vi "Run Test.vi"(8 "error in (no error)":errorcluster, 11 "Example Test In":refnum<class "Program RF.lvclass">) -> (0 "error out":errorcluster, 1 "Fail Codes":string[](array[string]), 2 "Tests Passed":bool[](array[boolean]), 3 "Example Test Out":refnum<class "Program RF.lvclass">)   [LabVIEW 2015, in "Program RF.lvclass"]
uses:
  Program RF.lvclass
  Test Class/Test Class.lvclass/Test Class.ctl
  <userlib>/_OpenG.lib/array/array.llb/Filter 1D Array with Scalar (Boolean)__ogtk.vi
  Classes/Application/Class/Application.lvclass
  Test Class/Test Class.lvclass
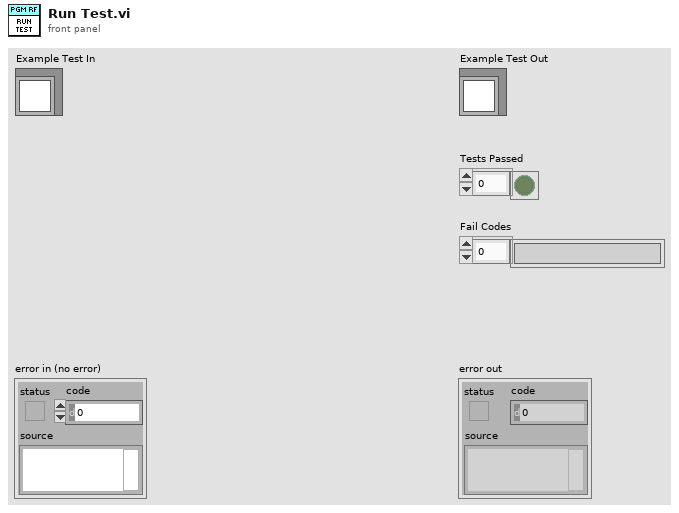
[diagram p1: front panel]
types:
  T1 = cluster{"status":bool, "code":i32, "source":string, "Position":u32}
  T2 = cluster{"Serial Number Reference":refnum<vi>, "Status Message Reference":refnum<vi>, "Position":u32}[]
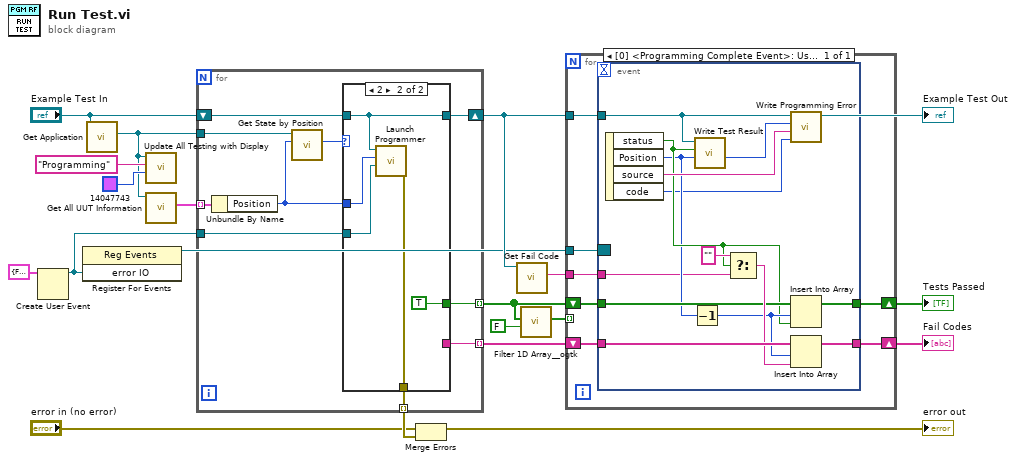
[diagram p0: block diagram]
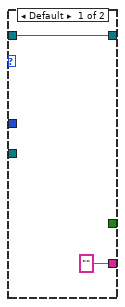
[diagram p2: hidden frame]
diagram:
  n1 = Create User Event(user event datatype=T1 {"status"=FALSE, "code"=0, "source"="", "Position"=0} ("error IO")) -> (user event=w1:refnum<user-event>)  [unwired: 1 in, 1 out]
  n2 = register-events(w1) -> (reference out=w4:refnum<event-registration>)  [unwired: 2 in, 1 out]
  n3 = call "Get Application.vi"("Test Class in"="Example Test In") -> ("Application.lvlib:Application.lvclass"=w3:refnum<class "Application.lvclass">)  [unwired: 9 in, 1 out]
  n4 = call "Update All Testing with Display.vi"("BG Color"=u32 14047743, "Message ('')"="Programming", "Application in"=w3) -> ()  [unwired: 7 in, 2 out]
  n5 = call-dynamic "Get All UUT Information.vi"("Application in"=w3) -> ("Active UUTs"=w15:T2)  [unwired: 8 in, 2 out]
  n6 = for {
    shift-right: [w25] -> w5
    shift-left: "Example Test In" -> [w27]
    tunnel: w15 -> [w29] mode=indexing
    tunnel: w3 -> [w24]
    tunnel: [w23] -> w10 mode=indexing
    tunnel: [w22] -> w14 mode=indexing
    tunnel: [w21] -> w13 mode=indexing
    tunnel: w1 -> [w20]
    n7 = Unbundle By Name(w29) -> ("Position"=w26:u32)
    n8 = call-dynamic "Get State by Position.vi"("Position"=w26, "Application in"=w24) -> ("State"=w28:u32)  [unwired: 7 in, 2 out]
    n9 = case shown="2" w28 {
      tunnel: w27 -> [w31 w33]
      tunnel: [w31 w33] -> w25
      tunnel: w26 -> [_ w36]
      tunnel: [_ TRUE] -> w23
      tunnel: ["" _] -> w22
      tunnel: [_ w34] -> w21
      tunnel: w20 -> [_ w32]
      frame Default {
      }
      frame 2 {
        n10 = call "Launch Programmer.vi"("Programming Complete Event"=w32, "Position"=w36, "Program RF in"=w33) -> ("error out"=w34:errorcluster)  [unwired: 8 in]
      }
    }
  }
  "Example Test Out" <- w5
  n11 = Merge Errors("error in (no error)", w13) -> (→"error out":errorcluster)
  n12 = call "Get Fail Code.vi"("Test Class in"=w5) -> ("Fail Code"=w6:string)  [unwired: 9 in, 1 out]
  n13 = call-poly <userlib>:"Filter 1D Array__ogtk.vi"("items to filter"=FALSE, "array"=w10) -> ("filtered array"=w9:bool[])  [unwired: 4 in, 1 out]
  n14 = for {
    tunnel: w4 -> [w43]
    shift-right: [w40] -> w18
    shift-left: w10 -> [w42]
    shift-right: [w39] -> w17
    shift-left: w14 -> [w41]
    tunnel: w9 -> [_] mode=indexing
    tunnel: w5 -> [w38]
    tunnel: w6 -> [w37]
    n15 = event shown="[0] <Programming Complete Event>: User Event" {
      selector: w43 -> [_]
      dyn-events: _ -> [_]
      timeout: _ -> [_]
      tunnel: w38 -> [w45]
      tunnel: w42 -> [w52]
      tunnel: w41 -> [w54]
      tunnel: [w49] -> w40
      tunnel: [w48] -> w39
      tunnel: w37 -> [w44]
      event User Event {
        n16 = event-data() -> ("status"=w50:bool, "Position"=w47:u32, "source"=w55:string, "code"=w46:i32)  [unwired: 1 in]
        n17 = Decrement(x=w47) -> (x-1=w51:u32)
        n18 = call "Write Test Result.vi"("Position"=w47, "Test Passed"=w50, "Test Class.lvclass"=w45) -> ()  [unwired: 9 in]
        n19 = Select(t="", s=w50, f=w44) -> (s? t:f=w53:string)
        n20 = call "Write Programming Error.vi"("code"=w46, "source"=w55, "Position"=w47, "Program RF in"=w45) -> ()  [unwired: 8 in]
        n21 = Insert Into Array(array=w52, index=w51, new element=w50) -> (w49:bool[])
        n22 = Insert Into Array(array=w54, index=w51, new element=w53) -> (w48:string[])
      }
    }
  }
  "Tests Passed" <- w18
  "Fail Codes" <- w17
